vi "openneodevice.vi"(4 "bSyncToPC? (F)":bool, 6 "bConfigRead? (T)":bool=TRUE, 8 "error in (no error)":errorcluster, 10 "bNetworkIDs":i8[](array[ring])=[0] items=["NETID_DEVICE"=0, "NETID_HSCAN"=1, "NETID_MSCAN"=2, "NETID_SWCAN"=3, "NETID_LSFTCAN"=4, "NETID_FORDSCP"=5, "NETID_J1708"=6, "NETID_AUX"=7, "NETID_JVPW"=8, "NETID_ISO_LIN"=9, "NETID_ISOPIC"=10, "NETID_MAIN51"=11, "NETID_SCI"=13, "NETID_ISO2"=14, "NETID_FIRE_HSCAN1"=41, "NETID_FIRE_HSCAN2"=42, "NETID_FIRE_MSCAN1"=43, "NETID_FIRE_MSCAN2_HSCAN3"=44, "NETID_FIRE_SWCAN"=45, "NETID_FIRE_LSFT"=46, "NETID_FIRE_LIN1"=47, "NETID_FIRE_LIN2"=48, "NETID_FIRE_LIN3"=49, "NETID_FIRE_LIN4"=50], 11 "NeoDevice{}":T1={"DeviceType"=65535, "Handle"=0, "NumberOfClients"=0, "SerialNumber"=0, "MaxAllowedClients"=0} {"DeviceType" items=["NEODEVICE_BLUE"=1, "NEODEVICE_DW_VCAN"=4, "NEODEVICE_FIRE"=8, "NEODEVICE_VCAN3"=16, "NEODEVICE_YELLOW"=32, "NEODEVICE_ALL"=65535]}) -> (0 "error out":errorcluster, 3 "hObject":i32)   [LabVIEW 2009]
doc: "this vi opens the port to the device\n\n<B>NeoDevices {}</B> : the device to be opened\n\n<B>bNetworkIDs</B> : the network IDs for each device. Wire \"0\" for the default ID.\n\n<B>bConfigRead? (T)</B> : whether to read the neoVI's device configuration before enabling the device. default is TRUE.\n\n<B>bSyncToPC? <F></B> : whether to synch the message time with the PC clock.\n\n<B>hObject</B> : the handle value of the neoVI driver object returned by the function call, it is to be used by other neoVI calls.\n\n12/21/2010 1.0.0 jyg\n- initial release"
uses:
  NEO VI Example/data/icsneo40.dll
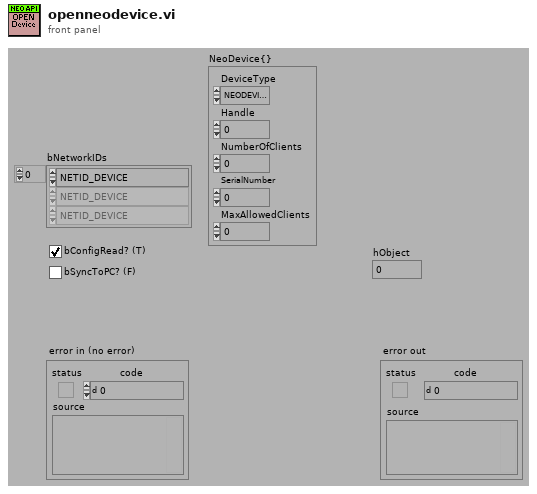
[diagram p1: front panel]
types:
  T1 = cluster{"DeviceType":i32, "Handle":i32, "NumberOfClients":i32, "SerialNumber":i32, "MaxAllowedClients":i32}
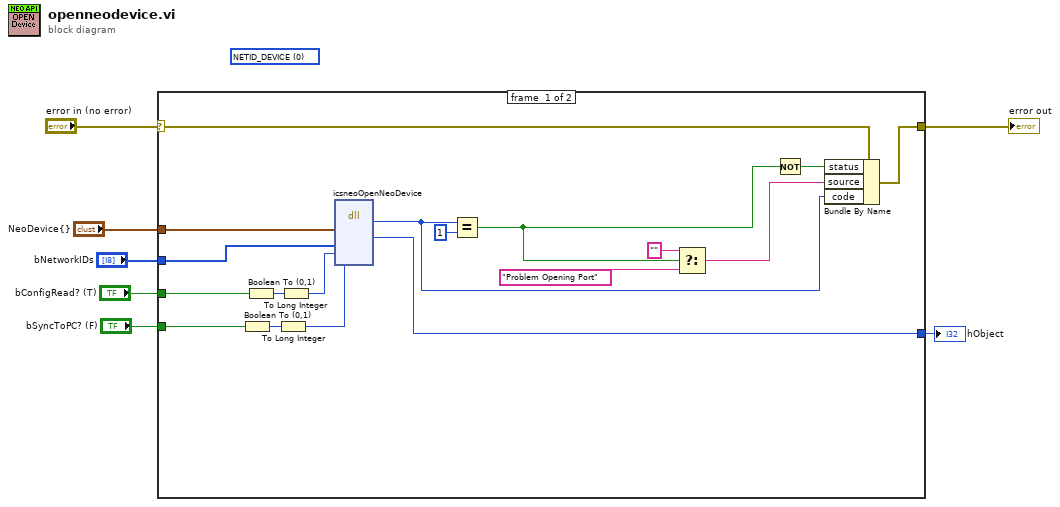
[diagram p0: block diagram]
diagram:
  (unwired) i8 0 items=["NETID_DEVICE"=0, "NETID_HSCAN"=1, "NETID_MSCAN"=2, "NETID_SWCAN"=3, "NETID_LSFTCAN"=4, "NETID_FORDSCP"=5, "NETID_J1708"=6, "NETID_AUX"=7, "NETID_JVPW"=8, "NETID_ISO_LIN"=9, "NETID_ISOPIC"=10, "NETID_MAIN51"=11, "NETID_SCI"=13, "NETID_ISO2"=14, "NETID_FIRE_HSCAN1"=41, "NETID_FIRE_HSCAN2"=42, "NETID_FIRE_MSCAN1"=43, "NETID_FIRE_MSCAN2_HSCAN3"=44, "NETID_FIRE_SWCAN"=45, "NETID_FIRE_LSFT"=46, "NETID_FIRE_LIN1"=47, "NETID_FIRE_LIN2"=48, "NETID_FIRE_LIN3"=49, "NETID_FIRE_LIN4"=50]
  n1 = case shown="No Error" "error in (no error)" {
    selector: "error in (no error)" -> [w22 w26]
    tunnel: [w23 w26] -> w7
    tunnel: "NeoDevice{}" -> [w21 _]
    tunnel: [w20 _] -> w4
    tunnel: "bNetworkIDs" -> [w19 _]
    tunnel: "bConfigRead? (T)" -> [w18 _]
    tunnel: "bSyncToPC? (F)" -> [w15 _]
    frame #0 {
      n2 = Boolean To (0,1)(Boolean=w15) -> (0, 1=w14:i16)
      n3 = Boolean To (0,1)(Boolean=w18) -> (0, 1=w17:i16)
      n4 = To Long Integer(number=w14) -> (32bit integer=w13:i32)
      n5 = To Long Integer(number=w17) -> (32bit integer=w16:i32)
      n6 = dll-call lib="C:/WINDOWS/system32/icsneo40.dll" fn="icsneoOpenNeoDevice"("NeoDevice"=w21, "bNetworkIDs"=w19, "bConfigRead"=w16, "bSyncToPC"=w13) -> ("return type"=w12:i32, "hObject"=w20:i32)  [unwired: 7 in, 3 out]
      n7 = Equal?(x=w12, y=1) -> (x = y?=w11:bool)
      n8 = Select(t="", s=w11, f="Problem Opening Port") -> (s? t:f=w8:string)
      n9 = Not(x=w11) -> (.not. x?=w24:bool)
      n10 = Bundle By Name(cluster=w22, "status"=w24, "source"=w8, "code"=w12) -> (w23:errorcluster)
    }
    frame #1 {
    }
  }
  "error out" <- w7
  "hObject" <- w4
